vi "VRMS_DC_Filter_compute_Rev01.vi"(0 "INPUT1 Data":dbl[](array[numeric]), 1 "L Input shift Shift V":dbl, 2 "L input multiplier":dbl, 3 "R Input multiplier":dbl, 5 "INPUT2 Data":dbl[](array[numeric]), 7 "Control Character":string, 9 "DC filter ON/OFF":bool, 11 "Number Of Samples":dbl, 13 "R Input Shift V":dbl) -> (4 "INPUT1 Vave":dbl, 6 "INPUT2 Vave":dbl, 10 "INPUT1RMS":dbl, 12 "INPUT1 Y array":dbl[](array[numeric]), 14 "INPUT2 Y array":dbl[](array[numeric]), 15 "INPUT2RMS":dbl)   [LabVIEW 2012]
panel:
  out "IN2R Mid":dbl[](graph)
  out "IN1L Mid":dbl[](graph)
  out "INPUT2R Line Out":dbl[](graph)
  out "INPUT1L Line Out":dbl[](graph)
  out "INPUT2R Line IN":dbl[](graph)
  out "INPUT1L Line IN":dbl[](graph)
  out "INPUT 1 in array":dbl[](array[numeric])
  # "WORK IN PROGRESS"
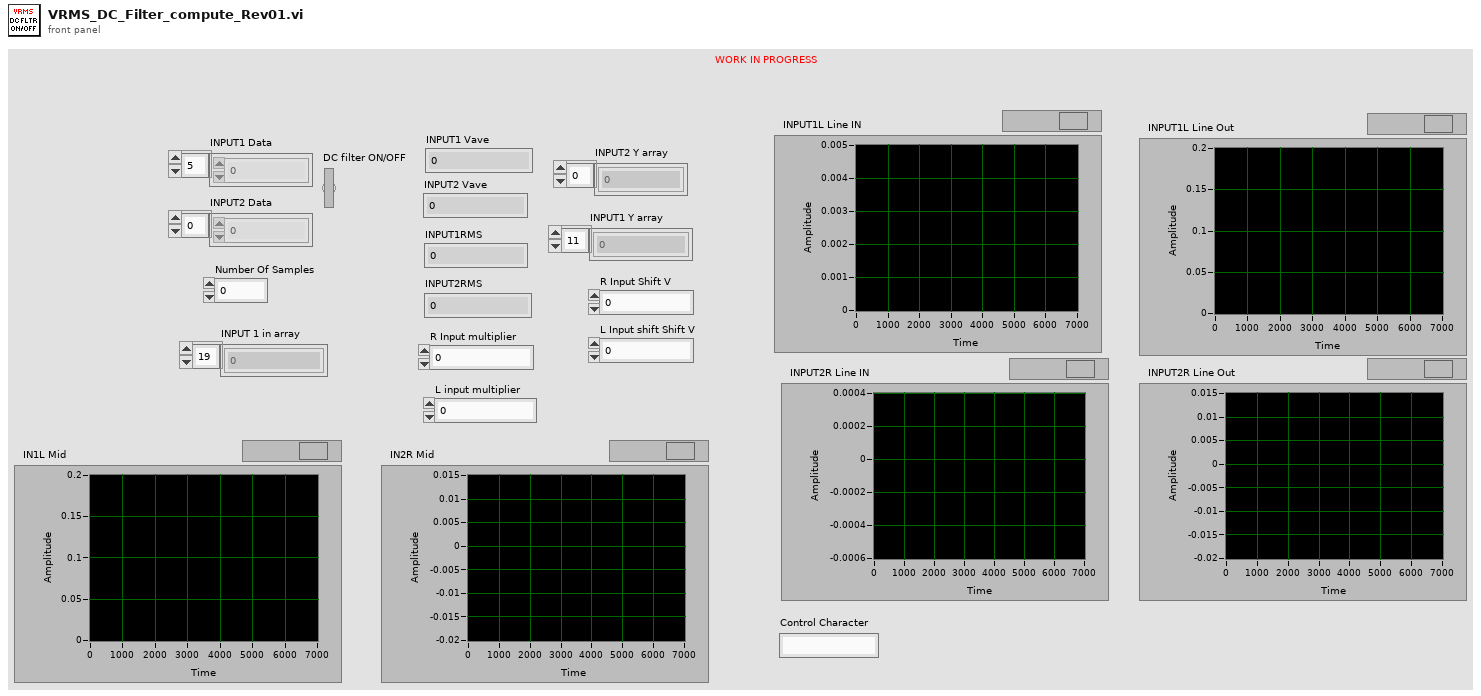
[diagram p1: front panel]
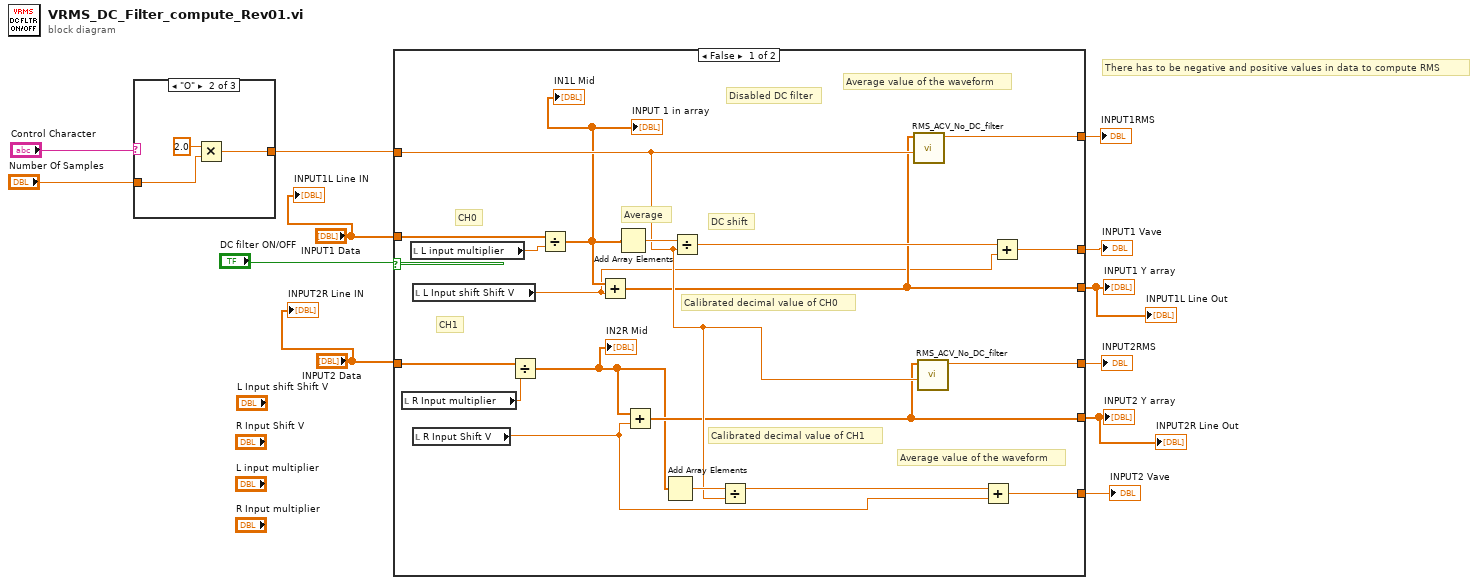
[diagram p0: block diagram]
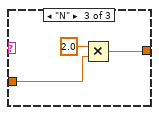
[diagram p3: hidden frame]
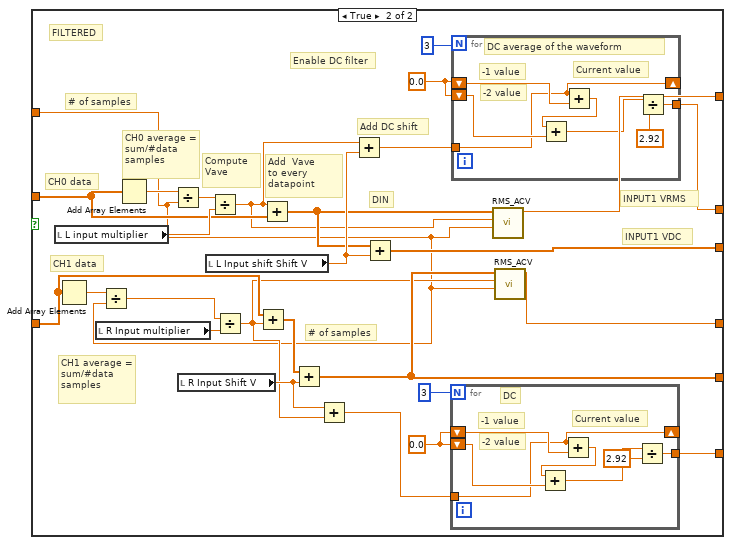
[diagram p4: hidden frame]
diagram:
  # "There has to be negative and positive values in data to compute RMS"
  n1 = case shown="\"O\"" "Control Character" {
    tunnel: [w13 w16 w18] -> w1
    tunnel: "Number Of Samples" -> [w13 w14 w17]
    frame "S", Default {
    }
    frame "O" {
      n2 = Multiply(x=2.0, y=w14) -> (x*y=w16:dbl)
    }
    frame "N" {
      n3 = Multiply(x=2.0, y=w17) -> (x*y=w18:dbl)
    }
  }
  n4 = case shown="False" "DC filter ON/OFF" {
    tunnel: "INPUT1 Data" -> [w35 w50]
    tunnel: "INPUT2 Data" -> [w38 w49]
    tunnel: [w26 w42] -> w5
    tunnel: [w27 w48] -> w4
    tunnel: [w29 w53] -> w9
    tunnel: [w31 w57] -> w11
    tunnel: w1 -> [w32 w40]
    tunnel: [w34 w43] -> w8
    tunnel: [w33 w39] -> w10
    frame False {
      # "CH1"
      # "CH0"
      # "Average value of the waveform"
      # "Average value of the waveform"
      # "Disabled DC filter"
      # "Calibrated decimal value of CH1"
      # "Calibrated decimal value of CH0"
      # "DC shift"
      # "Average"
      n5 = local read "R Input multiplier"() -> (w22:dbl)
      n6 = local read "L input multiplier"() -> (w23:dbl)
      n7 = local read "L Input shift Shift V"() -> (w20:dbl)
      n8 = local read "R Input Shift V"() -> (w21:dbl)
      n9 = Divide(x=w38, y=w22) -> (x/y=w25:dbl[])
      "IN2R Mid" <- w25
      n10 = Divide(x=w35, y=w23) -> (x/y=w24:dbl[])
      "INPUT 1 in array" <- w24
      "IN1L Mid" <- w24
      n11 = Add(x=w24, y=w20) -> (x+y=w27:dbl[])
      n12 = Add Array Elements(numeric array=w24) -> (sum=w37:dbl)
      n13 = Add(x=w25, y=w21) -> (x+y=w26:dbl[])
      n14 = Add Array Elements(numeric array=w25) -> (sum=w36:dbl)
      n15 = Divide(x=w37, y=w32) -> (x/y=w30:dbl)
      n16 = Divide(x=w36, y=w32) -> (x/y=w28:dbl)
      n17 = call "RMS_ACV_No_DC_filter.vi"("# of samples"=w32, "Data IN"=w27) -> ("VRMS"=w34:dbl)  [unwired: 9 in]
      n18 = call "RMS_ACV_No_DC_filter.vi"("# of samples"=w32, "Data IN"=w26) -> ("VRMS"=w33:dbl)  [unwired: 9 in]
      n19 = Add(x=w28, y=w21) -> (x+y=w29:dbl)
      n20 = Add(x=w30, y=w20) -> (x+y=w31:dbl)
    }
    frame True {
      w54 = 0.0
      w59 = 0.0
      # "DIN"
      # "Enable DC filter"
      # "FILTERED"
      # "CH1 average = sum/#data samples"
      # "INPUT1 VRMS"
      # "INPUT1 VDC"
      # "Add DC shift"
      # "Compute Vave"
      # "# of samples"
      # "# of samples"
      # "CH1 data"
      # "CH0 data"
      # "Add  Vave\nto every datapoint"
      # "CH0 average = sum/#data samples"
      n21 = local read "L input multiplier"() -> (w61:dbl)
      n22 = Add Array Elements(numeric array=w49) -> (sum=w64:dbl)
      n23 = local read "R Input multiplier"() -> (w60:dbl)
      n24 = Divide(x=w64, y=w40) -> (x/y=w63:dbl)
      n25 = Add Array Elements(numeric array=w50) -> (sum=w65:dbl)
      n26 = Divide(x=w65, y=w40) -> (x/y=w47:dbl)
      n27 = local read "R Input Shift V"() -> (w52:dbl)
      n28 = local read "L Input shift Shift V"() -> (w56:dbl)
      n29 = Divide(x=w47, y=w61) -> (x/y=w44:dbl)
      n30 = Divide(x=w63, y=w60) -> (x/y=w41:dbl)
      n31 = Add(x=w49, y=w41) -> (x+y=w62:dbl[])
      n32 = Add(x=w44, y=w50) -> (x+y=w45:dbl[])
      n33 = Add(x=w62, y=w52) -> (x+y=w42:dbl[])
      n34 = Add(x=w52, y=w41) -> (x+y=w51:dbl)
      n35 = Add(x=w44, y=w56) -> (x+y=w55:dbl)
      n36 = Add(x=w45, y=w56) -> (x+y=w48:dbl[])
      n37 = for {
        N: 3 -> [_]
        shift-right: [w66] -> _
        shift-left: w54 -> [w72]
        shift-left: w54 -> [w69]
        tunnel: [w67] -> w53
        tunnel: w51 -> [w66]
        # "DC"
        # "-2 value"
        # "-1 value"
        # "Current value"
        n38 = Add(x=w66, y=w72) -> (x+y=w70:dbl)
        n39 = Add(x=w70, y=w69) -> (x+y=w68:dbl)
        n40 = Divide(x=w68, y=2.92) -> (x/y=w67:dbl)
      }
      n41 = for {
        N: 3 -> [_]
        shift-right: [w73] -> _
        shift-left: w59 -> [w79]
        shift-left: w59 -> [w76]
        tunnel: [w74] -> w57
        tunnel: w55 -> [w73]
        # "DC average of the waveform"
        # "-2 value"
        # "-1 value"
        # "Current value"
        n42 = Add(x=w73, y=w79) -> (x+y=w77:dbl)
        n43 = Add(x=w77, y=w76) -> (x+y=w75:dbl)
        n44 = Divide(x=w75, y=2.92) -> (x/y=w74:dbl)
      }
      n45 = call "RMS_ACV.vi"("# of samples"=w40, "Vave"=w44, "Data IN"=w45) -> ("VRMS"=w43:dbl)  [unwired: 8 in]
      n46 = call "RMS_ACV.vi"("# of samples"=w40, "Vave"=w41, "Data IN"=w42) -> ("VRMS"=w39:dbl)  [unwired: 8 in]
    }
  }
  "INPUT1 Vave" <- w11
  "INPUT2 Vave" <- w9
  "INPUT1RMS" <- w8
  "INPUT2RMS" <- w10
  "INPUT2 Y array" <- w5
  "INPUT1 Y array" <- w4
  "INPUT1L Line Out" <- w4
  "INPUT2R Line Out" <- w5
  "INPUT2R Line IN" <- "INPUT2 Data"
  "INPUT1L Line IN" <- "INPUT1 Data"
